vi "SetCursorPos(ObjectName)diagram.vi"(6 "Relative x,y":T2, 7 "vi reference":refnum<vi>, 8 "error in (no error)":errorcluster, 9 "owner refnum":refnum<vi>, 10 "DesignCoreData":T1, 11 "name/order":string="While Loop") -> (0 "Error out":errorcluster, 2 "GObj Refnum":refnum<vi>, 3 "Sucess?":i32)   [LabVIEW 2013]
uses:
  <vilib>/Utility/miscctls.llb/LVPositionTypeDef.ctl
  Window VIs/DesignCoreData.ctl
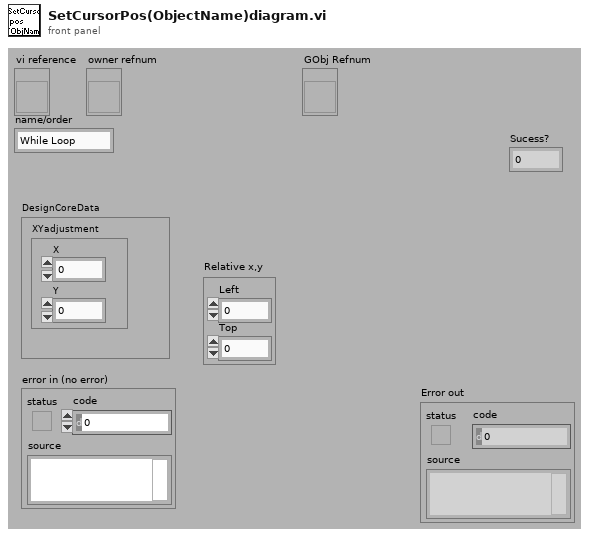
[diagram p1: front panel]
types:
  T1 = typedef "DesignCoreData.ctl" = cluster{"XYadjustment":cluster{"X":i32, "Y":i32}}
  T2 = typedef "LVPositionTypeDef.ctl" = cluster{"Left":i32, "Top":i32}
  T3 = typedef "LVRectTypeDef.ctl" = cluster{"Left":i16, "Top":i16, "Right":i16, "Bottom":i16}
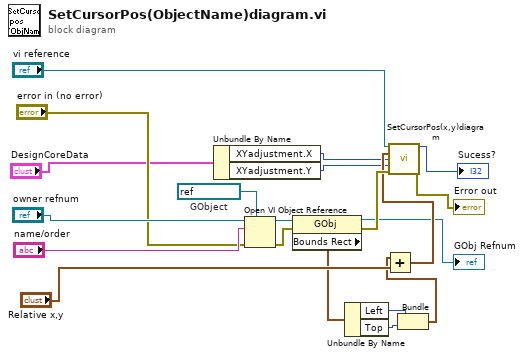
[diagram p0: block diagram]
diagram:
  w4 = refnum<vi> refnum  # GObject
  n1 = Unbundle By Name("DesignCoreData") -> ("XYadjustment.X"=w2:i32, "XYadjustment.Y"=w1:i32)
  n2 = Open VI Object Reference(7:w4, 8:"error in (no error)", 10:"name/order", 11:"owner refnum") -> (0:w17:errorcluster, 3:w18:refnum<vi>)
  n3 = property class="GObj"(reference=w18, error in=w17) -> (reference out=→"GObj Refnum":refnum<vi>, error out=w16:errorcluster, "Bounds Rect"=w8:T3)
  n4 = Unbundle By Name(w8) -> ("Left"=w7:i16, "Top"=w6:i16)
  n5 = Bundle("Left"=w7, "Top"=w6) -> (w5:cluster{"Left":i16, "Top":i16})  [unwired: 1 out]
  n6 = Add(x=w5, y="Relative x,y") -> (x+y=w12:T2)
  n7 = call "SetCursorPos(x,y)diagram.vi"("vi reference"="vi reference", "(X,Y)"=w12, "Xadjustment"=w2, "Yadjustment"=w1, "Error in"=w16) -> ("Sucess?"=→"Sucess?":i32, "Error out"=→"Error out":errorcluster)  [unwired: 9 out]
